vi "Teleop.vi"(10 "Match Info":T1={"Autonomous Elapsed Seconds"=0.0, "TeleOp Elapsed Seconds"=0.0, "Disabled Elapsed Seconds"=0.0, "Visited Autonomous"=FALSE, "Visited TeleOp"=FALSE, "Visited Disabled"=FALSE, "Autonomous Settings"={"Autonomous Style"=enum."Independent", "VI Refnum"=refnum}}, 11 "Call Context":T2) -> ()   [LabVIEW 2011]
doc: "This VI is called for each TeleOp packet received from the DS where the robot is not disabled. It is often used to read from the joysticks and update I/O or to update setpoints for timed control loops. It should complete and return within 20 milliseconds or it may miss DS packets."
uses:
  <vilib>/Rock Robotics/WPI/DriverStation/WPI_DriverStationDerivedRobotMode.ctl
  <vilib>/Rock Robotics/WPI/DriverStation/WPI_DriverStationMatch Info.ctl
  <vilib>/Rock Robotics/WPI/Relay/WPI_RelayValue.ctl
  Robot Global Data.vi
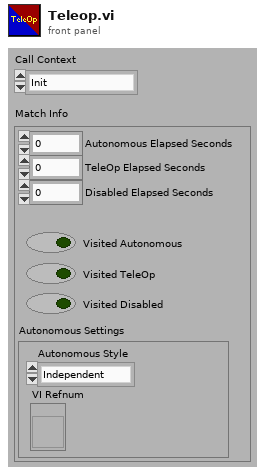
[diagram p1: front panel]
types:
  T1 = typedef "WPI_DriverStationMatch Info.ctl" = cluster{"Autonomous Elapsed Seconds":dbl, "TeleOp Elapsed Seconds":dbl, "Disabled Elapsed Seconds":dbl, "Visited Autonomous":bool, "Visited TeleOp":bool, "Visited Disabled":bool, "Autonomous Settings":cluster{"Autonomous Style":enum16{"Iterative", "Independent"}, "VI Refnum":refnum<vi>}}
  T2 = typedef "WPI_DriverStationDerivedRobotMode.ctl" = enum16{"Init", "Execute", "Stop"}
  T3 = typedef "WPI_RelayValue.ctl" = enum16{"Off", "On", "Forward", "Reverse"}
  T4 = typedef "WPI_JoystickDevRef.ctl" = cluster{"Device":T5}
  T5 = typedef "WPI_JoystickDeviceEnum.ctl" = enum16{"USB 1", "USB 2", "USB 3", "USB 4", "Kinect 1", "Kinect 2"}
  T6 = typedef "WPI_JoystickButtonState.ctl" = cluster{"Button 1":bool, "Button 2":bool, "Button 3":bool, "Button 4":bool, "Button 5":bool, "Button 6":bool, "Button 7":bool, "Button 8":bool, "Button 9":bool, "Button 10":bool, "Button 11":bool, "Button 12":bool}
  T7 = cluster{"axis 1 (x)":dbl, "axis 2 (y)":dbl, "axis 3 (throttle)":dbl, "axis 4":dbl, "axis 5":dbl, "axis 6":dbl}
  T8 = typedef "WPI_MotorControlDeviceRef.ctl" = cluster{"DeviceStatus":errorcluster, "Type":enum16{"PWM", "CAN"}, "PWM":cluster{"Digital Module":T9, "PWM Channel":T10, "DeadBand":T11}, "CAN":cluster{"Device Number":u8, "Control Mode":T12, "Semaphore":T13, "Max Vout":dbl}, "Invert":bool, "TransformRef":T14, "InvTransformRef":T14}
  T9 = typedef "FPGA_TypedefDigitalModule.ctl" = enum16{"Digital Module 1", "Digital Module 2"}
  T10 = typedef "FPGA_DIOPWMChannel.ctl" = enum8{"PWM 1", "PWM 2", "PWM 3", "PWM 4", "PWM 5", "PWM 6", "PWM 7", "PWM 8", "PWM 9", "PWM 10", "Invalid"}
  T11 = typedef "WPI_PWMDeadband.ctl" = cluster{"Name":string, "maxPositivePwm":i32, "minPositivePwm":i32, "centerPwm":i32, "maxNegativePwm":i32, "minNegativePwm":i32, "angularRange":u16}
  T12 = typedef "WPI_CANJaguar_ControlMode.ctl" = enum8{"Percent VBus", "Current", "Speed", "Position", "Voltage"}
  T13 = typedef "Semaphore RefNum" = refnum<k1>
  T14 = typedef "WPI_PWMTransform_ConPane.ctl" = refnum<vi>
  T15 = cluster{"Driver Station Digital Input (1-8)[0]":bool, "Driver Station Digital Input (1-8)[1]":bool, "Driver Station Digital Input (1-8)[2]":bool, "Driver Station Digital Input (1-8)[3]":bool, "Driver Station Digital Input (1-8)[4]":bool, "Driver Station Digital Input (1-8)[5]":bool, "Driver Station Digital Input (1-8)[6]":bool, "Driver Station Digital Input (1-8)[7]":bool, "Driver Station Digital Input (1-8)[8]":bool}
  T16 = typedef "WPI_RelayDevRef.ctl" = cluster{"DevStatus":errorcluster, "Relay Channel":T17, "Digital Module":T9, "Relay Direction":T18}
  T17 = typedef "FPGA_DIORelayChannel.ctl" = enum8{"Relay 1", "Relay 2", "Relay 3", "Relay 4", "Relay 5", "Relay 6", "Relay 7", "Relay 8", "Invalid"}
  T18 = typedef "WPI_RelayDirection.ctl" = enum16{"Both directions", "Forward only", "Reverse only"}
  T19 = typedef "WPI_DigitalInputDevRef.ctl" = cluster{"DevStatus":errorcluster, "DIO Channel":T20, "Digital Module":T9}
  T20 = typedef "FPGA_DIOChannel.ctl" = enum8{"DIO 1", "DIO 2", "DIO 3", "DIO 4", "DIO 5", "DIO 6", "DIO 7", "DIO 8", "DIO 9", "DIO 10", "DIO 11", "DIO 12", "DIO 13", "DIO 14", "Invalid"}
  T21 = typedef "WPI_RobotDriveDevRef.ctl" = cluster{"DevStatus":errorcluster, "Motors[]":T8[], "Square Inputs":bool, "Max Output":dbl, "Isochronous":bool}
  T22 = typedef "WPI_ServoDeviceRef.ctl" = cluster{"DeviceStatus":errorcluster, "Digital Module":T9, "PWM Channel":T10, "DeadBand":T11}
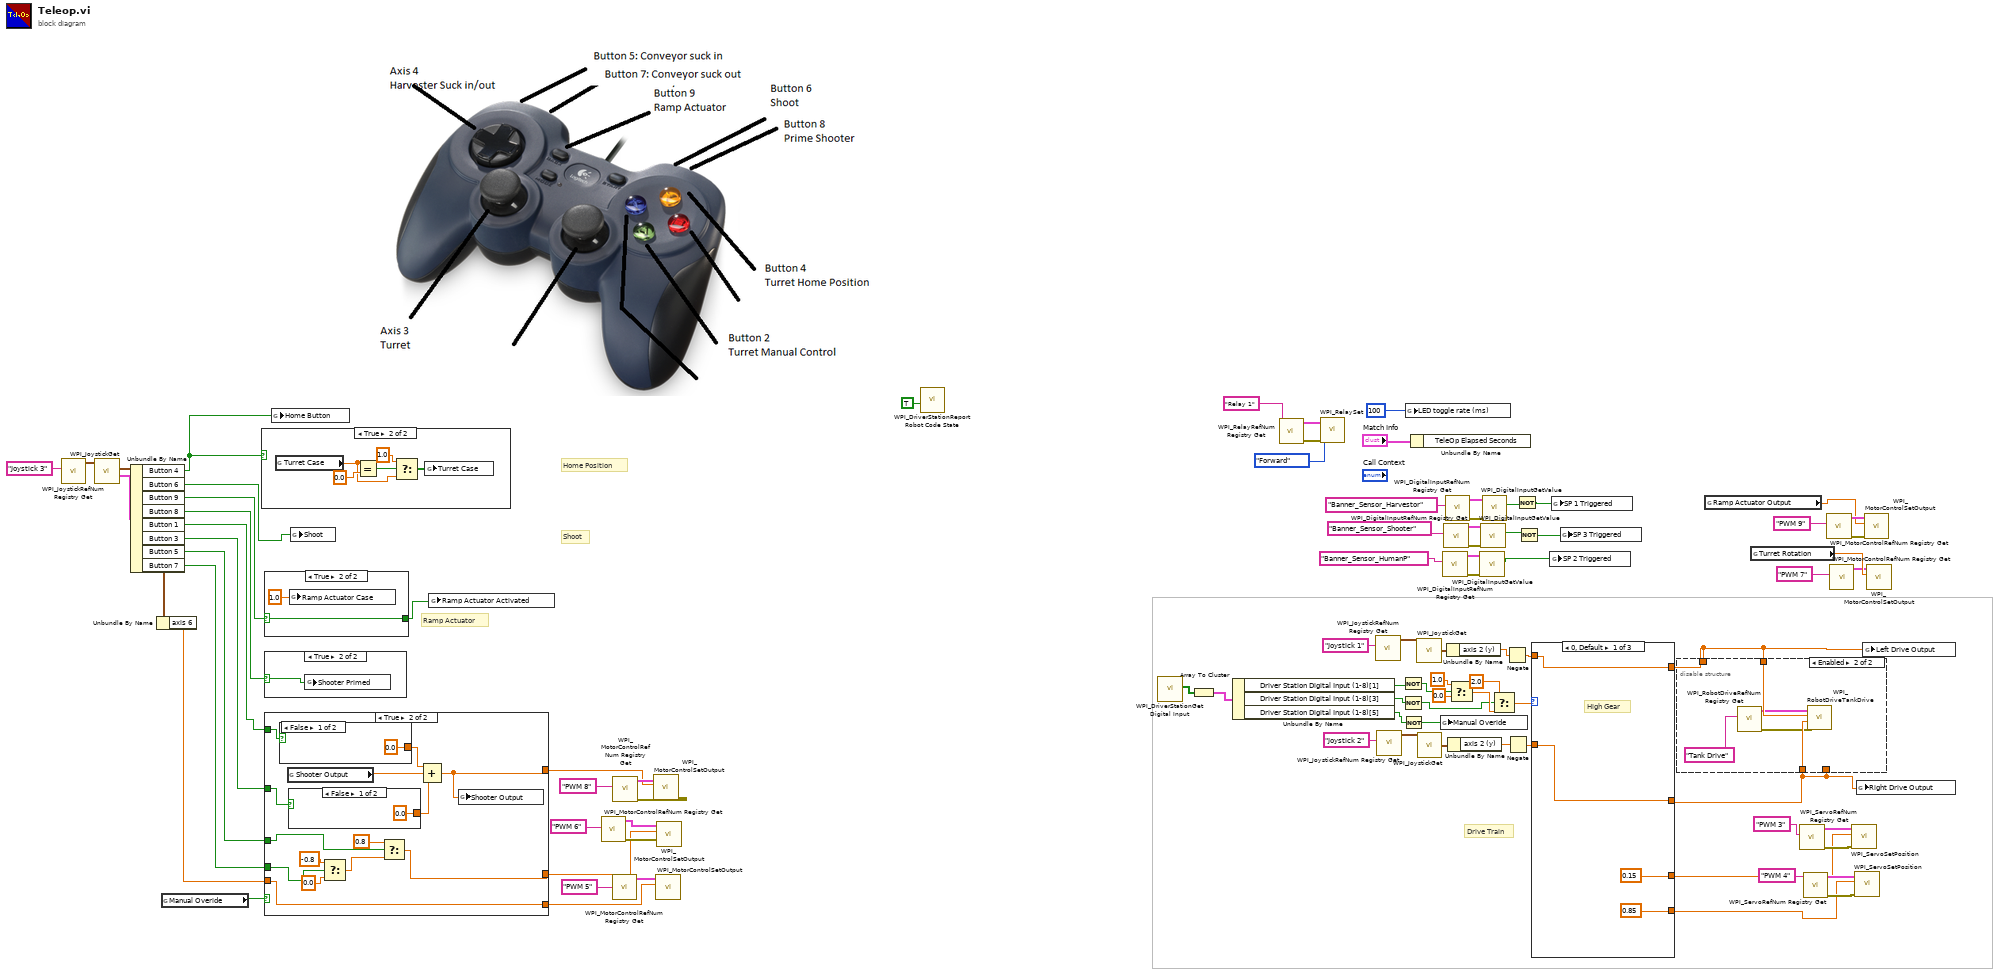
[diagram p0: block diagram]
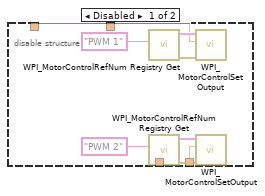
[diagram p2: hidden frame]
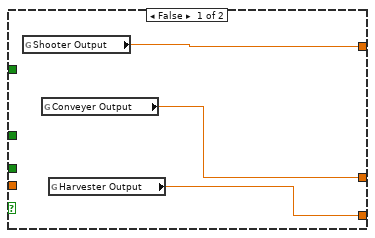
[diagram p3: hidden frame]
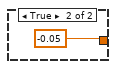
[diagram p4: hidden frame]
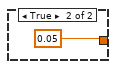
[diagram p5: hidden frame]
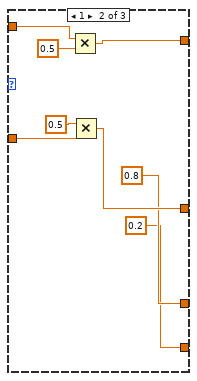
[diagram p9: hidden frame]
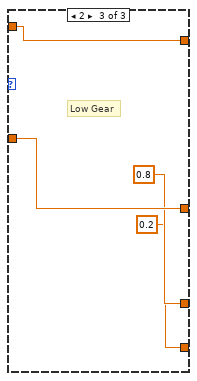
[diagram p10: hidden frame]
diagram:
  # "Home Position"
  # "Shoot"
  # "Ramp Actuator"
  # "Drive Train"
  n1 = call <vilib>:"WPI_JoystickRefNum Registry Get.vi"("refnum name"="Joystick 3") -> ("JoystickDevRef"=w47:T4)  [unwired: 9 in, 1 out]
  n2 = call <vilib>:"WPI_JoystickGet.vi"("JoystickDevRef"=w47) -> ("Buttons"=w48:T6, "Axes"=w19:T7)  [unwired: 4 in, 1 out]
  n3 = Unbundle By Name(w48) -> ("Button 4"=w46:bool, "Button 6"=w45:bool, "Button 9"=w44:bool, "Button 8"=w20:bool, "Button 1"=w14:bool, "Button 3"=w13:bool, "Button 5"=w12:bool, "Button 7"=w11:bool)
  n4 = Unbundle By Name(w19) -> ("axis 6"=w6:dbl)
  n5 = global read "Robot Global Data.vi" "Manual Overide"() -> (w5:bool)
  n6 = case shown="True" w46 {
    frame False {
    }
    frame True {
      n7 = global read "Robot Global Data.vi" "Turret Case"() -> (w89:dbl)
      n8 = Equal?(x=w89, y=0.0) -> (x = y?=w91:bool)
      n9 = Select(t=1.0, s=w91, f=w89) -> (s? t:f=w88:dbl)
      n10 = global write "Robot Global Data.vi" "Turret Case"(w88) -> ()
    }
  }
  n11 = case shown="True" w44 {
    selector: w44 -> [w93 w95]
    tunnel: [w93 w95] -> w50
    frame False {
    }
    frame True {
      n12 = global write "Robot Global Data.vi" "Ramp Actuator Case"(1.0 ("Ramp Actuator Case")) -> ()
    }
  }
  n13 = case shown="True" w20 {
    selector: w20 -> [_ w96]
    frame False {
    }
    frame True {
      n14 = global write "Robot Global Data.vi" "Shooter Primed"(w96) -> ()
    }
  }
  n15 = case shown="True" w5 {
    tunnel: [w99 w100] -> w15
    tunnel: w14 -> [_ w105]
    tunnel: w13 -> [_ w104]
    tunnel: w12 -> [_ w108]
    tunnel: w11 -> [_ w109]
    tunnel: [w97 w107] -> w7
    tunnel: w6 -> [_ w106]
    tunnel: [w98 w106] -> w4
    frame False {
      n16 = global read "Robot Global Data.vi" "Shooter Output"() -> (w99:dbl)
      n17 = global read "Robot Global Data.vi" "Conveyer Output"() -> (w97:dbl)
      n18 = global read "Robot Global Data.vi" "Harvester Output"() -> (w98:dbl)
    }
    frame True {
      n19 = case shown="False" w105 {
        tunnel: [0.0 0.05] -> w103
        frame False {
        }
        frame True {
        }
      }
      n20 = global read "Robot Global Data.vi" "Shooter Output"() -> (w101:dbl)
      n21 = case shown="False" w104 {
        tunnel: [0.0 -0.05] -> w102
        frame False {
        }
        frame True {
        }
      }
      n22 = Select(t=-0.8, s=w109, f=0.0) -> (s? t:f=w113:dbl)
      n23 = Select(t=0.8, s=w108, f=w113) -> (s? t:f=w107:dbl)
      n24 = Compound Arithmetic op=ADD(w103, w101, w102) -> (w100:dbl)
      n25 = global write "Robot Global Data.vi" "Shooter Output"(w100) -> ()
    }
  }
  n26 = global write "Robot Global Data.vi" "Home Button"(w46) -> ()
  n27 = global write "Robot Global Data.vi" "Shoot"(w45) -> ()
  n28 = global write "Robot Global Data.vi" "Ramp Actuator Activated"(w50) -> ()
  n29 = call <vilib>:"WPI_MotorControlRefNum Registry Get.vi"("refnum name"="PWM 6") -> ("error out"=w8:errorcluster, "MotorControlDevRef"=w9:T8)  [unwired: 9 in]
  n30 = call <vilib>:"WPI_MotorControlRefNum Registry Get.vi"("refnum name"="PWM 5") -> ("MotorControlDevRef"=w38:T8)  [unwired: 9 in, 1 out]
  n31 = call <vilib>:"WPI_MotorControlRefNum Registry Get.vi"("refnum name"="PWM 8") -> ("error out"=w22:errorcluster, "MotorControlDevRef"=w23:T8)  [unwired: 9 in]
  n32 = call <vilib>:"WPI_MotorControlSetOutput.vi"("error in (no error)"=w22, "Output"=w15, "MotorControlDevRef"=w23) -> ()  [unwired: 7 in, 2 out]
  n33 = call <vilib>:"WPI_MotorControlSetOutput.vi"("Output"=w4, "MotorControlDevRef"=w38) -> ()  [unwired: 8 in, 2 out]
  n34 = call <vilib>:"WPI_MotorControlSetOutput.vi"("error in (no error)"=w8, "Output"=w7, "MotorControlDevRef"=w9) -> ()  [unwired: 7 in, 2 out]
  n35 = call <vilib>:"WPI_DriverStationReport Robot Code State.vi"("TeleOp"=TRUE ("Autonomous")) -> ()  [unwired: 10 in, 1 out]
  n36 = call <vilib>:"WPI_DriverStationGet Digital Input.vi"() -> ("Driver Station Digital Input (1-8)"=w61:bool[])  [unwired: 11 in]
  n37 = Array To Cluster(array=w61) -> (cluster=w84:T15)
  n38 = Unbundle By Name(w84) -> ("Driver Station Digital Input (1-8)[1]"=w64:bool, "Driver Station Digital Input (1-8)[3]"=w63:bool, "Driver Station Digital Input (1-8)[5]"=w16:bool)
  n39 = call <vilib>:"WPI_RelayRefNum Registry Get.vi"("refnum name"="Relay 1") -> ("error out"=w42:errorcluster, "RelayDevRef"=w43:T16)  [unwired: 9 in]
  n40 = call <vilib>:"WPI_RelaySet.vi"("error in (no error)"=w42, "RelayValue"=WPI_RelayValue."Forward", "RelayDevRef"=w43) -> ()  [unwired: 7 in, 2 out]
  n41 = call <vilib>:"WPI_JoystickRefNum Registry Get.vi"("refnum name"="Joystick 1") -> ("JoystickDevRef"=w77:T4)  [unwired: 9 in, 1 out]
  n42 = call <vilib>:"WPI_JoystickRefNum Registry Get.vi"("refnum name"="Joystick 2") -> ("JoystickDevRef"=w74:T4)  [unwired: 9 in, 1 out]
  n43 = Not(x=w64) -> (.not. x?=w62:bool)
  n44 = Not(x=w63) -> (.not. x?=w18:bool)
  n45 = Not(x=w16) -> (.not. x?=w17:bool)
  n46 = global write "Robot Global Data.vi" "LED toggle rate (ms)"(u32 100 ("LED ms toggle rate")) -> ()
  n47 = Unbundle By Name("Match Info") -> ()  [unwired: 1 out]
  n48 = call <vilib>:"WPI_JoystickGet.vi"("JoystickDevRef"=w77) -> ("Axes"=w76:T7)  [unwired: 4 in, 2 out]
  n49 = call <vilib>:"WPI_JoystickGet.vi"("JoystickDevRef"=w74) -> ("Axes"=w75:T7)  [unwired: 4 in, 2 out]
  n50 = global write "Robot Global Data.vi" "Manual Overide"(w17) -> ()
  n51 = call <vilib>:"WPI_DigitalInputRefNum Registry Get.vi"("refnum name"="Banner_Sensor_HumanP") -> ("error out"=w33:errorcluster, "DigitalInputDevRef"=w32:T19)  [unwired: 9 in]
  n52 = call <vilib>:"WPI_DigitalInputRefNum Registry Get.vi"("refnum name"="Banner_Sensor_Shooter") -> ("error out"=w34:errorcluster, "DigitalInputDevRef"=w35:T19)  [unwired: 9 in]
  n53 = call <vilib>:"WPI_DigitalInputRefNum Registry Get.vi"("refnum name"="Banner_Sensor_Harvestor") -> ("error out"=w37:errorcluster, "DigitalInputDevRef"=w36:T19)  [unwired: 9 in]
  n54 = Unbundle By Name(w76) -> ("axis 2 (y)"=w60:dbl)
  n55 = Unbundle By Name(w75) -> ("axis 2 (y)"=w58:dbl)
  n56 = Select(t=1.0, s=w62, f=0.0 ("t")) -> (s? t:f=w81:dbl)
  n57 = call <vilib>:"WPI_DigitalInputGetValue.vi"("error in (no error)"=w33, "DigitalInputDevRef"=w32) -> ("Value"=w28:bool)  [unwired: 7 in, 2 out]
  n58 = call <vilib>:"WPI_DigitalInputGetValue.vi"("error in (no error)"=w34, "DigitalInputDevRef"=w35) -> ("Value"=w27:bool)  [unwired: 7 in, 2 out]
  n59 = call <vilib>:"WPI_DigitalInputGetValue.vi"("error in (no error)"=w37, "DigitalInputDevRef"=w36) -> ("Value"=w25:bool)  [unwired: 7 in, 2 out]
  n60 = Select(t=2.0, s=w18, f=w81) -> (s? t:f=w79:dbl)
  n61 = Negate(x=w60) -> (-x=w59:dbl)
  n62 = Negate(x=w58) -> (-x=w57:dbl)
  n63 = Not(x=w25) -> (.not. x?=w24:bool)
  n64 = Not(x=w27) -> (.not. x?=w26:bool)
  n65 = case shown="0, Default" w79 {
    tunnel: w57 -> [w121 w126 w133]
    tunnel: [w121 w127 w133] -> w2
    tunnel: [w120 w128 w132] -> w1
    tunnel: [0.15 ("LeftShifter_Pos") 0.8 0.8] -> w66
    tunnel: [0.85 0.2 ("LeftShifter_Pos") 0.2 ("LeftShifter_Pos")] -> w65
    tunnel: w59 -> [w120 w124 w132]
    frame 0, Default {
      # "High Gear"
    }
    frame 1 {
      n66 = Multiply(x=w124, y=0.5) -> (x*y=w128:dbl)
      n67 = Multiply(x=0.5 ("y"), y=w126) -> (x*y=w127:dbl)
    }
    frame 2 {
      # "Low Gear"
    }
  }
  n68 = global write "Robot Global Data.vi" "SP 2 Triggered"(w28) -> ()
  n69 = global write "Robot Global Data.vi" "SP 1 Triggered"(w24) -> ()
  n70 = global write "Robot Global Data.vi" "SP 3 Triggered"(w26) -> ()
  n71 = disable-structure shown="Enabled" {
    disable-tunnel: w1 -> [w135 _]
    disable-tunnel: w2 -> [w134 _]
    disable-tunnel: w2 -> [_ w146]
    disable-tunnel: w1 -> [_ w145]
    frame Disabled {
      n72 = call <vilib>:"WPI_MotorControlRefNum Registry Get.vi"("refnum name"="PWM 1") -> ("error out"=w139:errorcluster, "MotorControlDevRef"=w141:T8)  [unwired: 9 in]
      n73 = call <vilib>:"WPI_MotorControlRefNum Registry Get.vi"("refnum name"="PWM 2") -> ("error out"=w138:errorcluster, "MotorControlDevRef"=w137:T8)  [unwired: 9 in]
      n74 = call <vilib>:"WPI_MotorControlSetOutput.vi"("error in (no error)"=w139, "Output"=w135, "MotorControlDevRef"=w141) -> ()  [unwired: 7 in, 2 out]
      n75 = call <vilib>:"WPI_MotorControlSetOutput.vi"("error in (no error)"=w138, "Output"=w134, "MotorControlDevRef"=w137) -> ()  [unwired: 7 in, 2 out]
    }
    frame Enabled {
      n76 = call <vilib>:"WPI_RobotDriveRefNum Registry Get.vi"("refnum name"="Tank Drive") -> ("error out"=w143:errorcluster, "RobotDriveDevRef"=w142:T21)  [unwired: 9 in]
      n77 = call <vilib>:"WPI_RobotDriveTankDrive.vi"("error in (no error)"=w143, "Right axis value"=w146, "Left axis value"=w145, "RobotDriveDevRef"=w142) -> ()  [unwired: 6 in, 2 out]
    }
  }
  n78 = global read "Robot Global Data.vi" "Ramp Actuator Output"() -> (w3:dbl)
  n79 = global read "Robot Global Data.vi" "Turret Rotation"() -> (w53:dbl)
  n80 = call <vilib>:"WPI_ServoRefNum Registry Get.vi"("refnum name"="PWM 3") -> ("error out"=w70:errorcluster, "ServoDeviceRef"=w71:T22)  [unwired: 9 in]
  n81 = call <vilib>:"WPI_ServoRefNum Registry Get.vi"("refnum name"="PWM 4") -> ("error out"=w69:errorcluster, "ServoDeviceRef"=w68:T22)  [unwired: 9 in]
  n82 = call <vilib>:"WPI_MotorControlRefNum Registry Get.vi"("refnum name"="PWM 9") -> ("error out"=w55:errorcluster, "MotorControlDevRef"=w54:T8)  [unwired: 9 in]
  n83 = call <vilib>:"WPI_MotorControlRefNum Registry Get.vi"("refnum name"="PWM 7") -> ("MotorControlDevRef"=w51:T8)  [unwired: 9 in, 1 out]
  n84 = call <vilib>:"WPI_ServoSetPosition.vi"("error in (no error)"=w70, "Position"=w66, "ServoDeviceRef"=w71) -> ()  [unwired: 7 in, 2 out]
  n85 = call <vilib>:"WPI_ServoSetPosition.vi"("error in (no error)"=w69, "Position"=w65, "ServoDeviceRef"=w68) -> ()  [unwired: 7 in, 2 out]
  n86 = global write "Robot Global Data.vi" "Right Drive Output"(w2) -> ()
  n87 = global write "Robot Global Data.vi" "Left Drive Output"(w1) -> ()
  n88 = call <vilib>:"WPI_MotorControlSetOutput.vi"("error in (no error)"=w55, "Output"=w3, "MotorControlDevRef"=w54) -> ()  [unwired: 7 in, 2 out]
  n89 = call <vilib>:"WPI_MotorControlSetOutput.vi"("Output"=w53, "MotorControlDevRef"=w51) -> ()  [unwired: 8 in, 2 out]
